vi "Load Stage dotnet control.vi"(8 "error in (no error)":errorcluster) -> (0 "error out":errorcluster, 1 "Long Travel Stage":refnum<k24>, 2 "Tools.wpf":refnum<k24>)   [LabVIEW 2020]
uses:
  C:/GEECS/Developers Version/builds/Device builds/ThorLabsLTS/Thorlabs.MotionControl.Controls.dll
  Thorlabs.MotionControl.Controls.dll
  C:/GEECS/Developers Version/builds/Device builds/ThorLabsLTS/Thorlabs.MotionControl.Tools.WPF.UI.dll
  Thorlabs.MotionControl.Tools.WPF.UI.dll
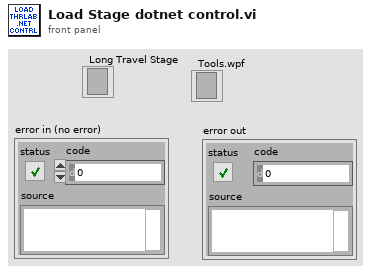
[diagram p1: front panel]
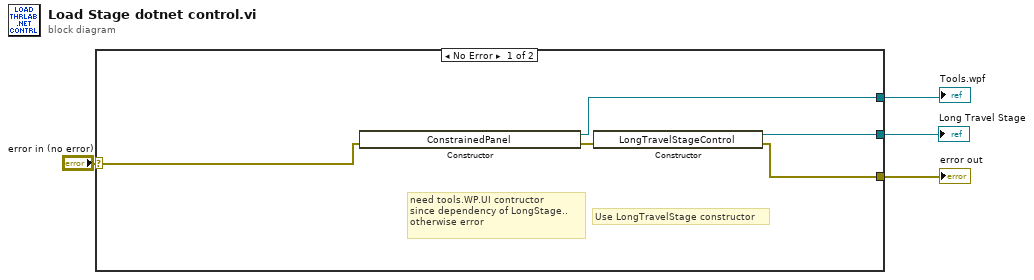
[diagram p0: block diagram]
diagram:
  n1 = case shown="No Error" "error in (no error)" {
    selector: "error in (no error)" -> [w7 w10]
    tunnel: [w8 _] -> w4
    tunnel: [w6 _] -> w2
    tunnel: [w5 w10] -> w1
    frame No Error {
      # "need tools.WP.UI contructor \nsince dependency of LongStage..\notherwise error"
      # "Use LongTravelStage constructor"
      n2 = constructor class="Thorlabs.MotionControl.Tools.WP"(error in=w7) -> (reference out=w6:refnum<k24>, error out=w9:errorcluster)  [unwired: 2 in, 1 out]
      n3 = constructor class="LongTravelStageControl"(error in=w9) -> (reference out=w8:refnum<k24>, error out=w5:errorcluster)  [unwired: 2 in, 1 out]
    }
    frame Error {
    }
  }
  "Long Travel Stage" <- w4
  "Tools.wpf" <- w2
  "error out" <- w1
